vi "split_modes_vec.vi"(11 "Decoupled":sgl[](array[numeric]) format="%#.0f") -> (0 "Rz":sgl, 1 "Z":sgl, 2 "Rx Ry":sgl[](array[numeric]), 3 "XY":sgl[](array[numeric]))   [LabVIEW 2013]
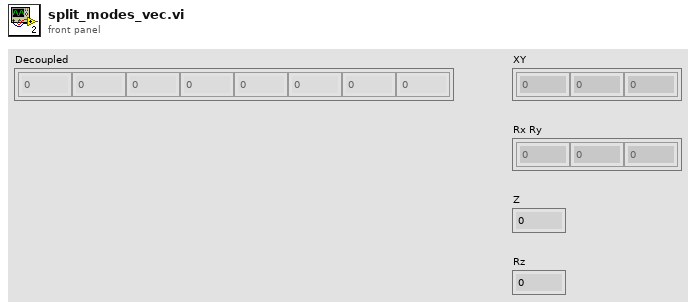
[diagram p1: front panel]
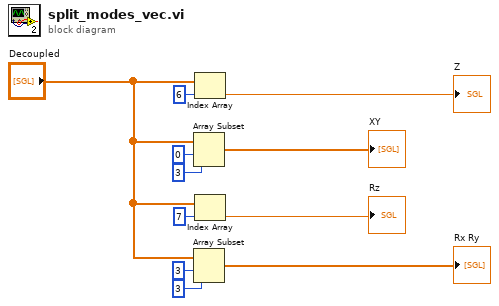
[diagram p0: block diagram]
diagram:
  n1 = Array Subset(array="Decoupled", index=0, length=3) -> (→"XY":sgl[])
  n2 = Array Subset(array="Decoupled", index=3, length=3) -> (→"Rx Ry":sgl[])
  n3 = Index Array(array="Decoupled", index=6) -> (element=→"Z":sgl)
  n4 = Index Array(array="Decoupled", index=7) -> (element=→"Rz":sgl)
